vi "addScripEvent.vi"(8 "error in (no error)":errorcluster, 10 "ScriptEvent":refnum<class "ScriptEvent.lvclass">, 11 "device in":refnum<class "device.lvclass">) -> (0 "error out":errorcluster, 3 "device out":refnum<class "device.lvclass">)   [LabVIEW 2011, in "Tools.lvlib" / "DatabaseHelpers.lvlib" / "device.lvclass"]
uses:
  device.lvclass
  Scripting/ScriptingEvent/ScriptEvent.lvclass
  device.lvclass/device.ctl
  Scripting/ScriptingEvent/ScriptEventList/ScriptEventList.lvclass
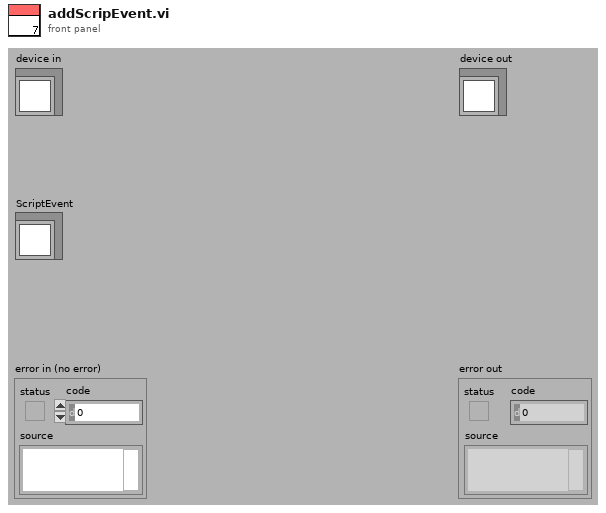
[diagram p1: front panel]
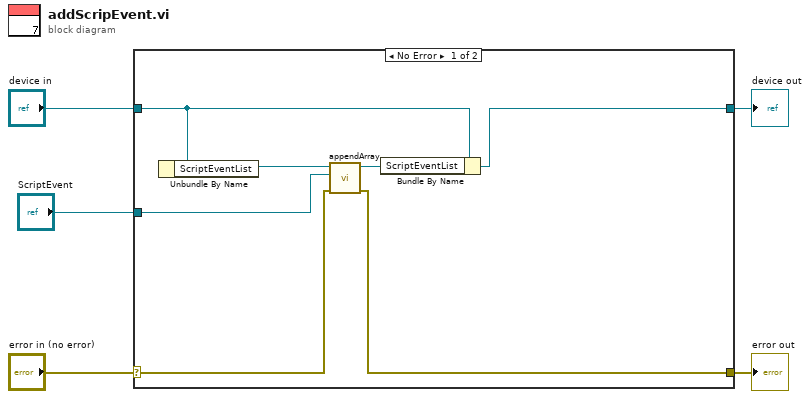
[diagram p0: block diagram]
diagram:
  n1 = case shown="No Error" "error in (no error)" {
    selector: "error in (no error)" -> [w10 w14]
    tunnel: [w9 w14] -> w4
    tunnel: [w6 w13] -> w2
    tunnel: "device in" -> [w7 w13]
    tunnel: "ScriptEvent" -> [w11 _]
    frame No Error {
      n2 = Unbundle By Name(w7) -> ("ScriptEventList"=w12:refnum<class "ScriptEventList.lvclass">)
      n3 = call "appendArray.vi"("error in (no error)"=w10, "ScriptEvent"=w11, "ScriptEventList in"=w12) -> ("error out"=w9:errorcluster, "ScriptEventList out"=w8:refnum<class "ScriptEventList.lvclass">)  [unwired: 6 in, 1 out]
      n4 = Bundle By Name(cluster=w7, "ScriptEventList"=w8) -> (w6:refnum<class "device.lvclass">)
    }
    frame Error {
    }
  }
  "error out" <- w4
  "device out" <- w2
